vi "Write Waveform to FPGA.vi"() -> ()   [LabVIEW 2015]
uses:
  <vilib>/Platform/TimedLoop/XDataNode/timing_clust.ctl
  <vilib>/Platform/TimedLoop/XDataNode/nitl_modes.ctl
  <vilib>/Platform/TimedLoop/XDataNode/wakeup.ctl
  <vilib>/rvi/Emulation/niFpgaGetClockAttributes.vi
  <vilib>/rvi/Emulation/niFpgaSctlEmulationGetInTimedLoop.vi
  <vilib>/rvi/Emulation/niFpgaEmulationReportErrorSimple.vi
  <vilib>/rvi/DataTransferAndStorage/Container/Common/niFpgaContainerExecOnDevCompGetState.vi
  <vilib>/rvi/Emulation/niFpgaEmulationIsFPGAContextNoSignature.vi
  <vilib>/rvi/errors/niFpgaSetErrorForExecOnDevCompSimple.vi
  <vilib>/rvi/eio/common/nirviEmuReportErrorAndStop.vi
  <vilib>/rvi/DataTransferAndStorage/Container/Common/niFpgaContainerGetUniqueNameForEmu.vi
  <vilib>/rvi/FIFO/Fifo_Resource/nirvififoEmulationSetSize.vi
  <vilib>/rvi/FIFO/Fifo_Resource/nirviFifoEmulationQueueMgr.vi
  <instcachedir>/0/nirviFifoEmulationQueueMgr_E5CAEC123FF24DC58D834DCA3CDAA9B5.lvgen/nirviFifoEmulationQueueMgr_E5CAEC123FF24DC58D834DCA3CDAA9B5_014.vi
  <vilib>/rvi/FIFO/Fifo_Resource/nirvififoEmulationDetermineInputValidOut.vi
  <vilib>/rvi/FIFO/Fifo_Resource/nirvififoEmulationCreateLock.vi
  <vilib>/rvi/Emulation/niFpgaProcessEmulError.vi
  <vilib>/rvi/FIFO/Fifo_Resource/nirvififoEmulationObtainLock.vi
  <vilib>/rvi/FIFO/Fifo_Resource/nirvififoEmulationReleaseLock.vi
  <vilib>/rvi/occurrence/nirviWaitOnOccurrenceBase.vi
  <vilib>/rvi/errors/nirviReportUnexpectedCaseInternalError.vi
  <vilib>/rvi/errors/nirviReportUnexpectedCaseInternalError (U32).vi
  <vilib>/Utility/error.llb/Clear Errors.vi
  <vilib>/rvi/interface/RandomDataEmulation/niFpgaRandomDataHandleErrors.vi
  <vilib>/rvi/Emulation/niFpgaCriticalErrorInLSC.vi
  <vilib>/rvi/Memory/Memory_Emulation/niFpgaMemoryEmulationDramWriteAndRequestDataApplyByteEnables.vi
  <vilib>/rvi/Memory/Memory_Emulation/niFpgaMemoryEmulationCacheClearOnFirstRun.vi
  <vilib>/rvi/Memory/Memory_Emulation/nirvimemoryEmulationManagerCache_MakeExclusive.vi
  <vilib>/rvi/Memory/Memory_Emulation/nirvimemoryEmulationManagerCache_GetValue.vi
  <vilib>/rvi/Memory/Memory_Emulation/nirvimemoryEmulationManagerCache_InsertValue.vi
  <vilib>/rvi/Memory/Memory_Emulation/nirvimemoryEmulationManagerCache_ReleaseExclusive.vi
  <vilib>/rvi/Memory/Memory_Emulation/nirvimemoryEmulationManagerCache_SetValue.vi
  <vilib>/Platform/TimedLoop/XDataNode/XDataNode.xnode
  <vilib>/rvi/DataTransferAndStorage/Container/XNode/niFpgaContainer.xnode
  <vilib>/rvi/FIFO/Fifo_Resource/niFpgaFifoEmulationRefIn.vi
  <vilib>/rvi/Memory/Memory_Emulation/niFpgaMemoryEmulationDramWriteAndRequestDataRefIn.vi
  <vilib>/rvi/Memory/Memory_Emulation/niFpgaMemoryEmulationDramRetrieveDataRefIn.vi
  <vilib>/Platform/TimedLoop/XDataNode/XDNodeRunTimeDep.lvlib
panel:
  out "wave points read":i32
  out "Max request address":u32
  out "Max wave DRAM address":u32
  out "Request Done":bool
  out "Read Done":bool
  out "Write Done":bool
  in  "Current Process":enum16{"Wait", "Write", "Read", "Stop"}(ring)
  in  "U16*32":u16[](array[numeric])=[0, 0, 0, 0, 0, 0, 0, 0, 0, 0, 0, 0, 0, 0, 0, 0, 0, 0, 0, 0, 0, 0, 0, 0, 0, 0, 0, 0, 0, 0, 0, 0]
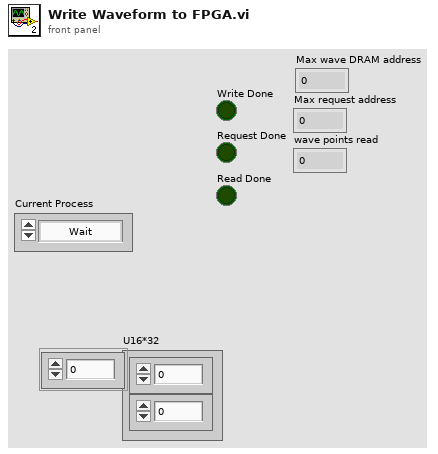
[diagram p1: front panel]
types:
  T1 = typedef "XDNodeRunTimeDep.lvlib/timing_clust.ctl" = cluster{"Expected End [f-1]":u64, "Actual End [f-1]":u64, "Finished Late? [f-1]":bool, "Expected End [i-1]":u64, "Actual End [i-1]":u64, "Finished Late? [i-1]":bool, "Expected Start [i]":u64, "Actual Start [i]":u64, "Expected Start [f]":u64, "Actual Start [f]":u64, "Source Name":string, "Structure Name":string, "Period":i64, "Deadline":i64, "Offset":i64, "Start":i64, "Priority":i32, "Timeout":i32, "Mode":T2, "Wakeup Reason":T3, "Error":errorcluster, "Source Type":string, "Secondary Source Type":string, "Global End Time":u64, "Global Start Time":u64, "Frame Duration":u64, "Iteration Duration":u64, "Assigned CPU":i32, "I/O Scan Engine Mode":u32}
  T2 = typedef "XDNodeRunTimeDep.lvlib/nitl_modes.ctl" = enum32{"No Change", "Process missed periods, maintain original phase", "Discard missed periods, maintain original phase", "Process missed periods, ignore original phase", "Discard missed periods, ignore original phase"}
  T3 = typedef "XDNodeRunTimeDep.lvlib/wakeup.ctl" = enum32{"Normal", "Aborted", "Asynchronous wakeup", "Timing source error", "Timed loop error", "Timeout"}
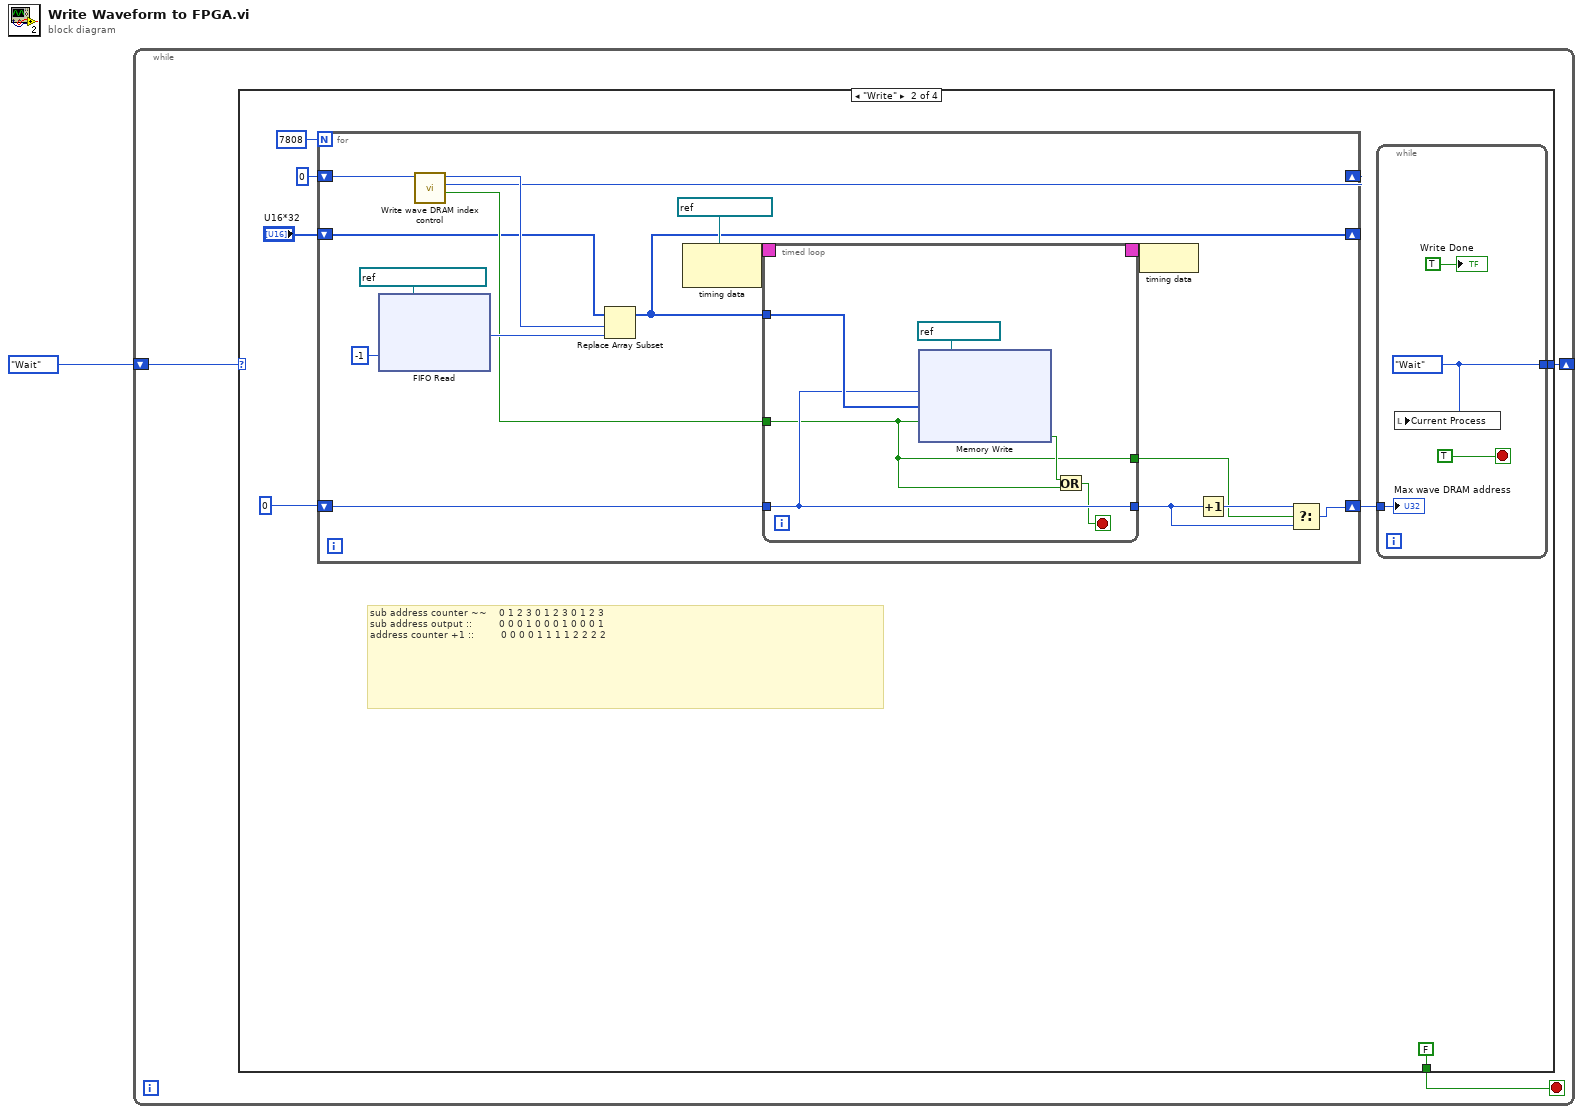
[diagram p0: block diagram]
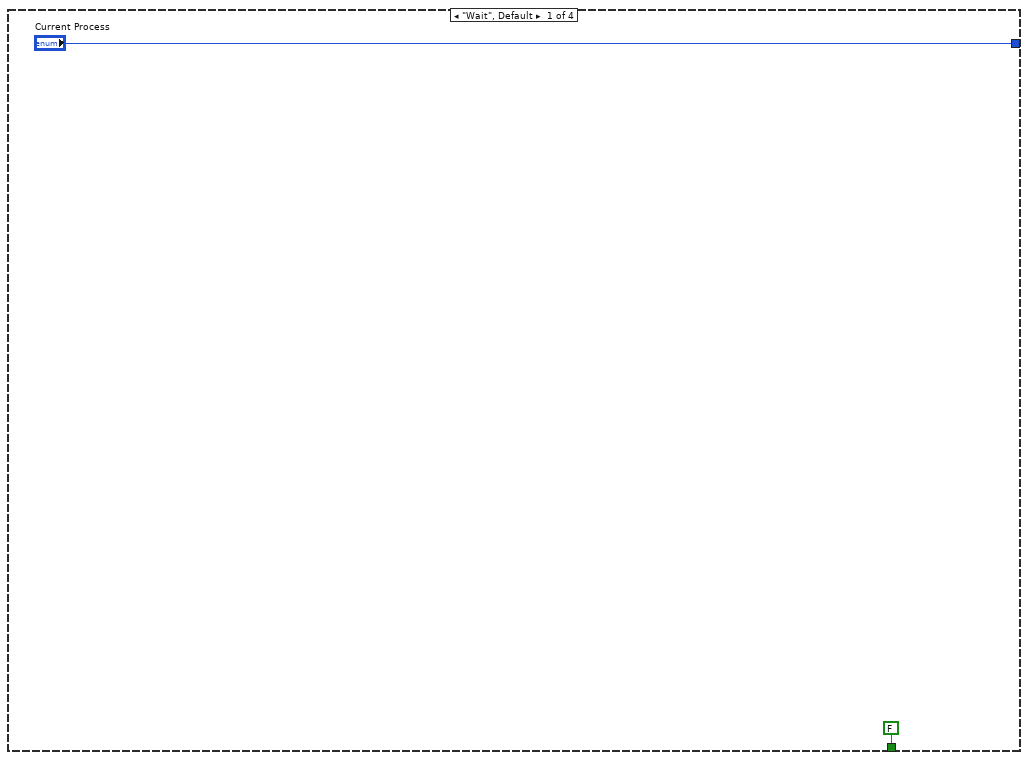
[diagram p2: hidden frame]
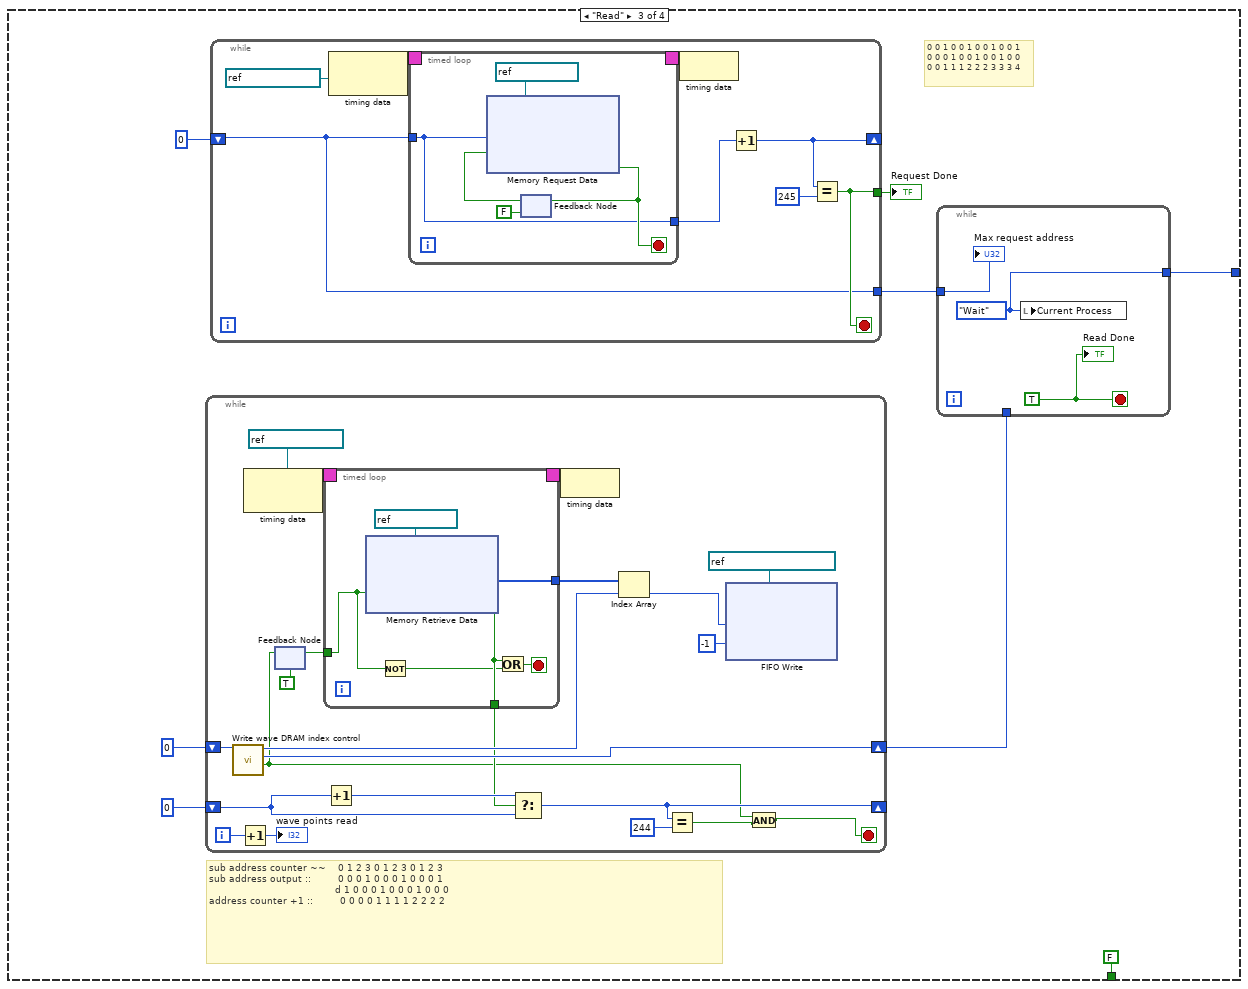
[diagram p3: hidden frame]
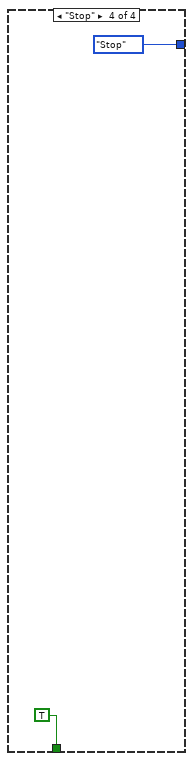
[diagram p4: hidden frame]
diagram:
  n1 = while {
    shift-right: [w4] -> _
    shift-left: enum16{"Wait", "Write", "Read", "Stop"}."Wait" -> [w3]
    stop <- w2 stop-if-true
    n2 = case shown="\"Write\"" w3 {
      tunnel: ["Current Process" w11 w50 enum16{"Wait", "Write", "Read", "Stop"}."Stop" ("Current Process")] -> w4
      tunnel: [FALSE FALSE FALSE TRUE] -> w2
      frame "Wait", Default {
      }
      frame "Write" {
        # "sub address counter ~~    0 1 2 3 0 1 2 3 0 1 2 3\nsub address output ::         0 0 0 1 0 0 0 1 0 0 0 1   \naddress counter +1 ::         0 0 0 0 1 1 1 1 2 2 2 2"
        n3 = for {
          N: 7808 -> [_]
          shift-right: [w22] -> w10
          shift-left: u32 0 ("地址") -> [w24]
          shift-right: [w27] -> _
          shift-left: 0 ("Next index") -> [w28]
          shift-right: [w18] -> _
          shift-left: "U16*32" -> [w19]
          n4 = xnode ("FIFO Read")("Timeout"=-1 ("超时"), "FIFO In"=refnum<k21> "Host to Target U16" ("FIFO输入")) -> ("Element"=w31:u16)  [unwired: 2 out]
          n5 = call "Write wave DRAM index control.vi"("Current index"=w28) -> ("Output Valid"=w26:bool, "Next index"=w27:i32, "Current index"=w30:i32)  [unwired: 8 in]
          n6 = Replace Array Subset(array=w19, new element=w31, index=w30) -> (w18:u16[])
          n7 = node-c288(refnum<k21> "DRAM Clock" ("源名称")) -> (w34:T1)
          n8 = timed-loop {
            timing: w34 -> [_]
            timing-out: [_] -> w33
            tunnel: w18 -> [w39]
            tunnel: w24 -> [w38]
            tunnel: [w38] -> w20
            tunnel: w26 -> [w35]
            tunnel: [w35] -> w21
            stop <- w37 stop-if-true
            n9 = xnode ("Memory Write")("Address"=w38, "Data"=w39, "Input Valid"=w35, "Memory In"=refnum<k21> "Waveform" ("存储器输入")) -> ("Ready for Input"=w36:bool)  [unwired: 1 out]
            n10 = Or(x=w36, y=w35) -> (x .or. y?=w37:bool)
          }
          n11 = node-c288(w33) -> ()
          n12 = Increment(x=w20) -> (x+1=w23:u32)
          n13 = Select(t=w23, s=w21, f=w20) -> (s? t:f=w22:u32)
        }
        n14 = while {
          tunnel: [w17] -> w11
          tunnel: w10 -> [w14]
          stop <- TRUE stop-if-true
          w17 = enum16{"Wait", "Write", "Read", "Stop"}."Wait"
          n15 = local write "Current Process"(w17) -> ()
          "Write Done" <- TRUE ("Write Done")
          "Max wave DRAM address" <- w14
        }
      }
      frame "Read" {
        # "0 0 1 0 0 1 0 0 1 0 0 1\n0 0 0 1 0 0 1 0 0 1 0 0\n0 0 1 1 1 2 2 2 3 3 3 4"
        # "sub address counter ~~    0 1 2 3 0 1 2 3 0 1 2 3\nsub address output ::         0 0 0 1 0 0 0 1 0 0 0 1  \n                                          d 1 0 0 0 1 0 0 0 1 0 0 0 \naddress counter +1 ::         0 0 0 0 1 1 1 1 2 2 2 2"
        n16 = while {
          shift-right: [w89] -> w51
          shift-left: 0 ("Current index") -> [w94]
          shift-right: [w86] -> _
          shift-left: 0 ("Current index") -> [w87]
          i -> [w81]
          stop <- w78 stop-if-true
          n17 = call "Write wave DRAM index control.vi"("Current index"=w94) -> ("Output Valid"=w80:bool, "Next index"=w89:i32, "Current index"=w93:i32)  [unwired: 8 in]
          n18 = Increment(x=w81) -> (x+1=→"wave points read":i32)
          n19 = node-c288(refnum<k21> "DRAM Clock" ("源名称")) -> (w98:T1)
          n20 = feedback-in #1(w80) -> ()
          n21 = feedback #1(TRUE ("Output Valid")) -> (w83:bool)
          n22 = timed-loop {
            timing: w98 -> [_]
            timing-out: [_] -> w97
            tunnel: [w103] -> w95
            tunnel: [w101] -> w84
            tunnel: w83 -> [w100]
            stop <- w102 stop-if-true
            n23 = xnode ("Memory Retrieve Data")("Ready for Output"=w100, "Memory In"=refnum<k21> "Waveform" ("存储器输入")) -> ("Data"=w103:u16[], "Output Valid"=w101:bool)  [unwired: 1 out]
            n24 = Not(x=w100) -> (.not. x?=w99:bool)
            n25 = Or(x=w101, y=w99) -> (x .or. y?=w102:bool)
          }
          n26 = Increment(x=w87) -> (x+1=w88:i32)
          n27 = Select(t=w88, s=w84, f=w87) -> (s? t:f=w86:i32)
          n28 = node-c288(w97) -> ()
          n29 = Index Array(array=w95, index=w93) -> (element=w91:u16)
          n30 = Equal?(x=w86, y=244) -> (x = y?=w79:bool)
          n31 = xnode ("FIFO Write")("Element"=w91, "Timeout"=-1 ("超时"), "FIFO In"=refnum<k21> "Target to Host U16" ("FIFO输入")) -> ()  [unwired: 2 out]
          n32 = And(x=w80, y=w79) -> (x .and. y?=w78:bool)
        }
        n33 = while {
          shift-right: [w57] -> _
          shift-left: u32 0 ("地址") -> [w55]
          tunnel: [w56] -> w48
          tunnel: [w55] -> w47
          stop <- w56 stop-if-true
          n34 = node-c288(refnum<k21> "DRAM Clock" ("源名称")) -> (w62:T1)
          n35 = timed-loop {
            timing: w62 -> [_]
            timing-out: [_] -> w61
            tunnel: w55 -> [w64]
            tunnel: [w64] -> w58
            stop <- w65 stop-if-true
            n36 = feedback #2(FALSE ("输入就绪")) -> (w63:bool)
            n37 = xnode ("Memory Request Data")("Address"=w64, "Input Valid"=w63, "Memory In"=refnum<k21> "Waveform" ("存储器输入")) -> ("Ready for Input"=w65:bool)  [unwired: 1 out]
            n38 = feedback-in #2(w65) -> ()
          }
          n39 = node-c288(w61) -> ()
          n40 = Increment(x=w58) -> (x+1=w57:u32)
          n41 = Equal?(x=w57, y=u32 245) -> (x = y?=w56:bool)
        }
        "Request Done" <- w48
        n42 = while {
          tunnel: w51 -> [_]
          tunnel: [w75] -> w50
          tunnel: w47 -> [w74]
          stop <- w76 stop-if-true
          w75 = enum16{"Wait", "Write", "Read", "Stop"}."Wait" ("Current Process")
          w76 = TRUE
          n43 = local write "Current Process"(w75) -> ()
          "Read Done" <- w76
          "Max request address" <- w74
        }
      }
      frame "Stop" {
      }
    }
  }
